vi "Clear_Ctrl_Watch_List.vi"(10 "Control Array":bool[][](array[boolean]), 11 "QuWire in":refnum<class "QuWire.lvclass">) -> (3 "QuWire out":refnum<class "QuWire.lvclass">)   [LabVIEW 2020, in "QuWire.lvclass"]
uses:
  QuWire.lvclass
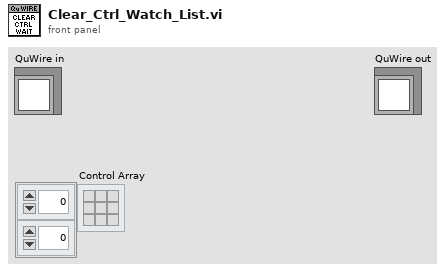
[diagram p1: front panel]
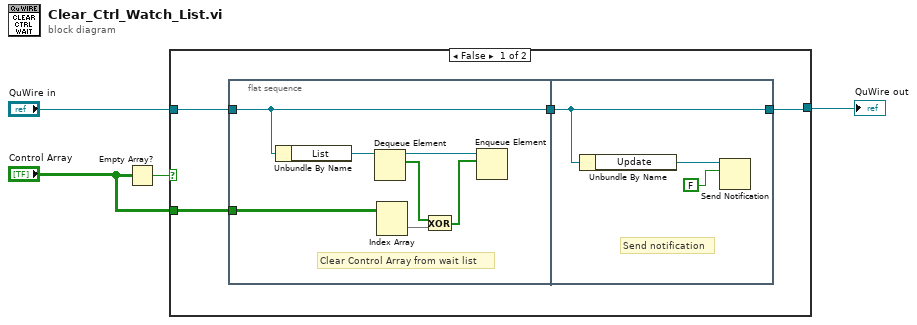
[diagram p0: block diagram]
diagram:
  n1 = Empty Array?(array="Control Array") -> (empty?=w1:bool)
  n2 = case shown="False" w1 {
    tunnel: "QuWire in" -> [w7 w19]
    tunnel: [w6 w19] -> w4
    tunnel: "Control Array" -> [w8 _]
    frame False {
      n3 = flat-sequence {
        tunnel: w8 -> [w10]
        tunnel: w7 -> [w9]
        tunnel: [w9] -> w5
        tunnel: [w18] -> w6
        tunnel: w5 -> [w18]
        frame #0 {
          # "Clear Control Array from wait list"
          n4 = Unbundle By Name(w9) -> ("List"=w12:refnum<queue>)
          n5 = Dequeue Element(queue=w12) -> (queue out=w14:refnum<queue>, element=w15:bool[])  [unwired: 2 in, 2 out]
          n6 = Index Array(array=w10) -> (element=w11:bool[])  [unwired: 2 in]
          n7 = Exclusive Or(1:w11, 2:w15) -> (0:w13:bool[])
          n8 = Enqueue Element(queue=w14, element=w13) -> ()  [unwired: 2 in, 3 out]
        }
        frame #1 {
          # "Send notification"
          n9 = Unbundle By Name(w18) -> ("Update"=w17:refnum<notifier>)
          n10 = Send Notification(notification=FALSE, notifier=w17) -> ()  [unwired: 1 in, 2 out]
        }
      }
    }
    frame True {
    }
  }
  "QuWire out" <- w4
